vi "eip_read.vi"(7 "error in":errorcluster, 10 "GPIB":refnum<visa-resource-name>) -> (0 "error out":errorcluster, 1 "read buffer":string, 2 "bytes returned":u32, 3 "VISA Resource Out":refnum<visa-resource-name>)   [LabVIEW 2018]
panel:
  out "Rsrc Name":string
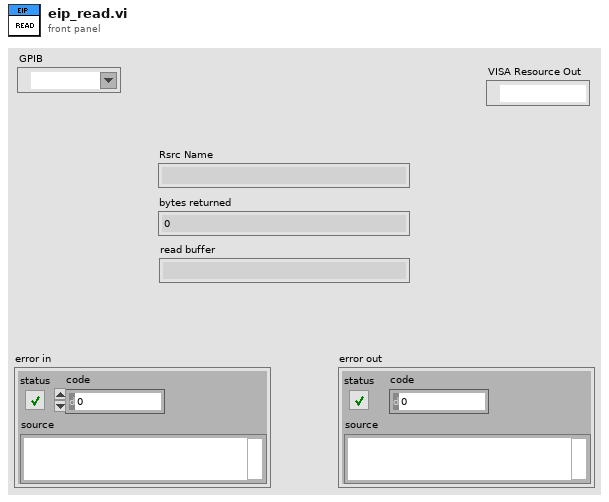
[diagram p1: front panel]
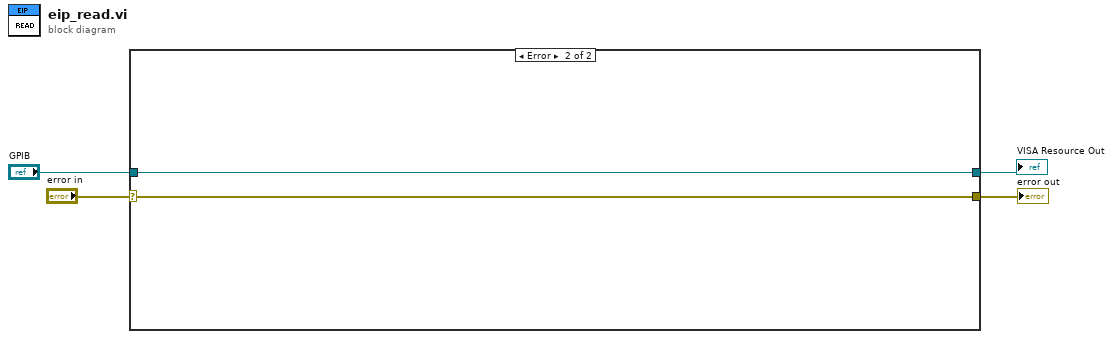
[diagram p0: block diagram]
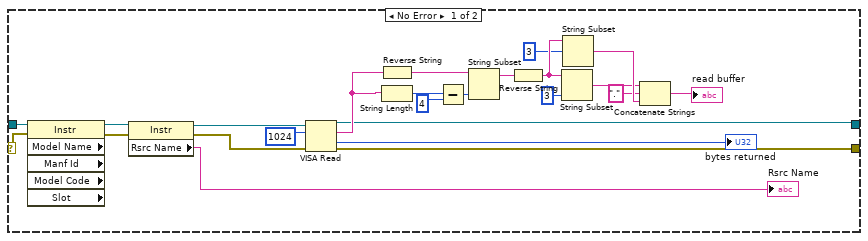
[diagram p2: hidden frame]
diagram:
  n1 = case shown="Error" "error in" {
    selector: "error in" -> [w6 w29]
    tunnel: "GPIB" -> [w22 w30]
    tunnel: [w7 w29] -> w3
    tunnel: [w5 w30] -> w1
    frame No Error {
      n2 = property class="Instr" props=["Model Name", "Manf Id", "Model Code", "Slot"](reference=w22, error in=w6) -> (reference out=w24:refnum<visa-resource-name>, error out=w25:errorcluster)  [unwired: 4 out]
      n3 = property class="Instr"(reference=w24, error in=w25) -> (reference out=w26:refnum<visa-resource-name>, error out=w27:errorcluster, "Rsrc Name"=→"Rsrc Name":string)
      n4 = VISA Read(VISA resource name=w26, byte count=u32 1024, error in (no error)=w27) -> (VISA resource name out=w5:refnum<visa-resource-name>, read buffer=w10:string, return count=→"bytes returned":u32, error out=w7:errorcluster)
      n5 = Reverse String(1:w10) -> (0:w9:string)
      n6 = String Length(string=w10) -> (length=w20:i32)
      n7 = Subtract(x=w20, y=4) -> (x-y=w18:i32)
      n8 = String Subset(string=w9, length (rest)=w18) -> (substring=w17:string)  [unwired: 1 in]
      n9 = Reverse String(1:w17) -> (0:w15:string)
      n10 = String Subset(string=w15, length (rest)=3 ("length (rest)")) -> (substring=w12:string)  [unwired: 1 in]
      n11 = String Subset(string=w15, offset (0)=3) -> (substring=w13:string)  [unwired: 1 in]
      n12 = Concatenate Strings(w12, "." ("string"), w13) -> (→"read buffer":string)
    }
    frame Error {
    }
  }
  "error out" <- w3
  "VISA Resource Out" <- w1
